vi "Match VI Names in String.vi"(10 "Application:All VIs In Memory":string[](array[string]), 11 "string":string) -> (3 "vi names":T1(array[cluster]))   [LabVIEW 2020, in "Explain Error Improved Dialog.lvlib"]
uses:
  Explain Error Improved Dialog/Explain Error Improved Dialog.lvlib
  <vilib>/regexp/Match Regular Expression.xnode
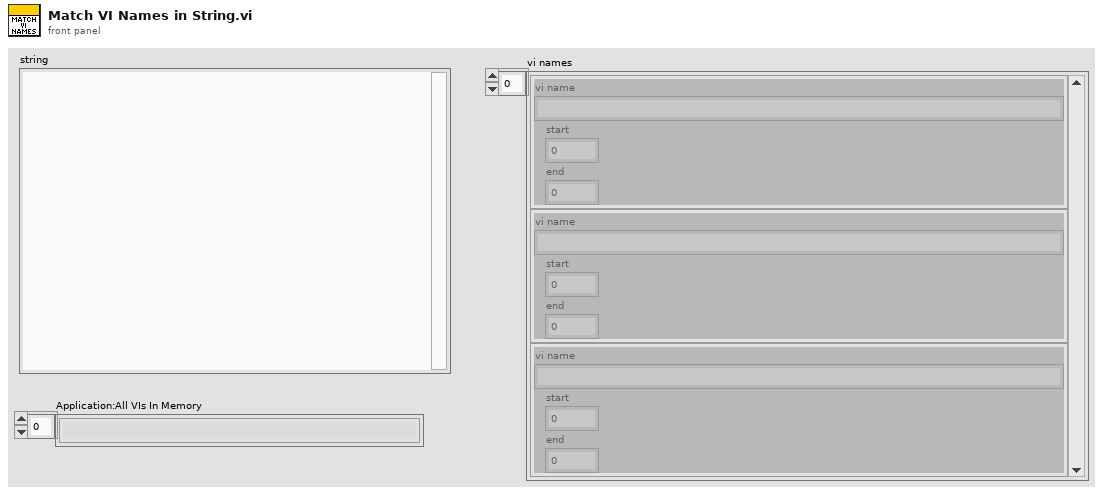
[diagram p1: front panel]
types:
  T1 = cluster{"vi name":string, "start":i32, "end":i32}[]
  T2 = cluster{"vi name":string, "start":i32, "end":i32}
  T3 = cluster{"submatch":string, "start":i32, "end":i32}
  T4 = cluster{"submatch":string, "start":i32, "end":i32}[]
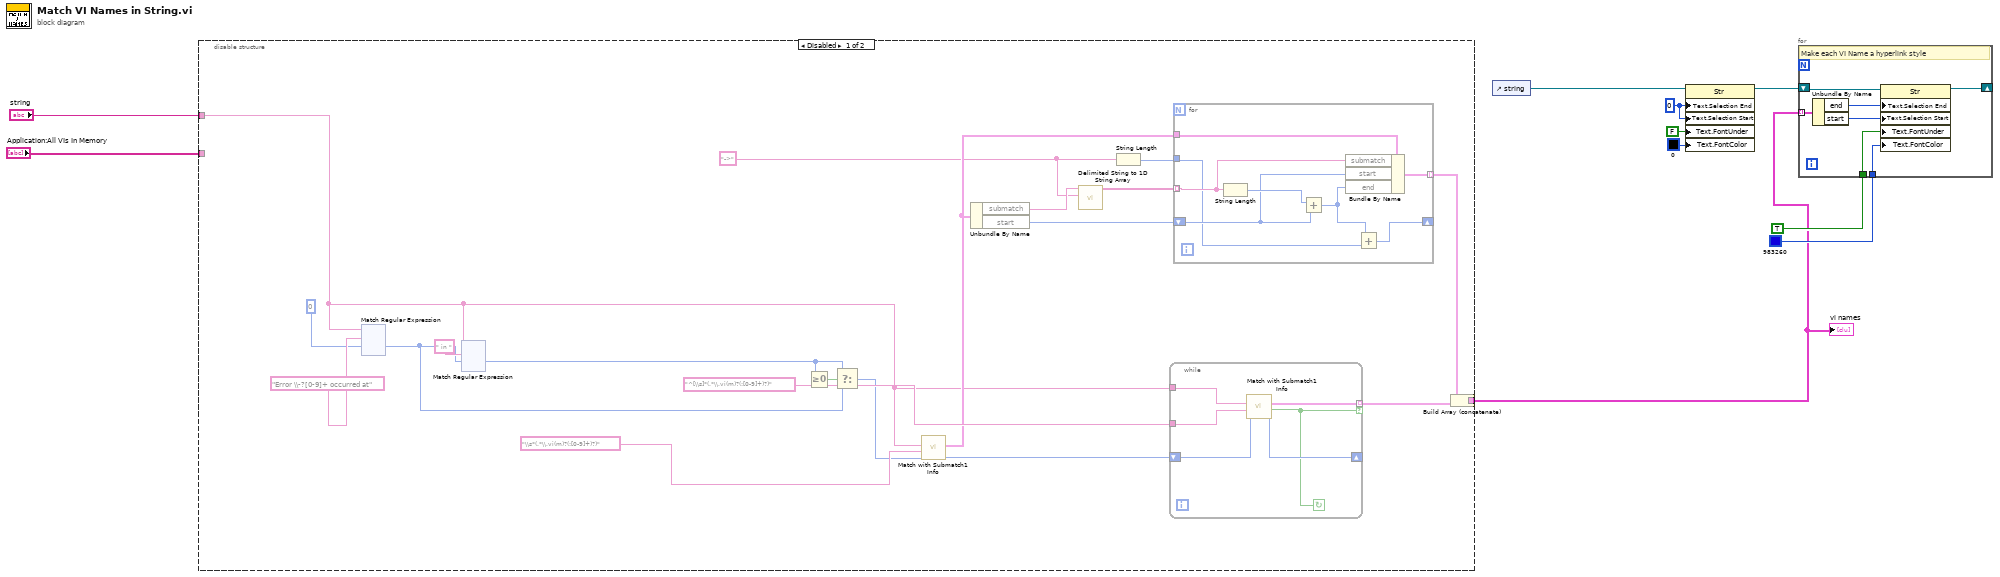
[diagram p0: block diagram]
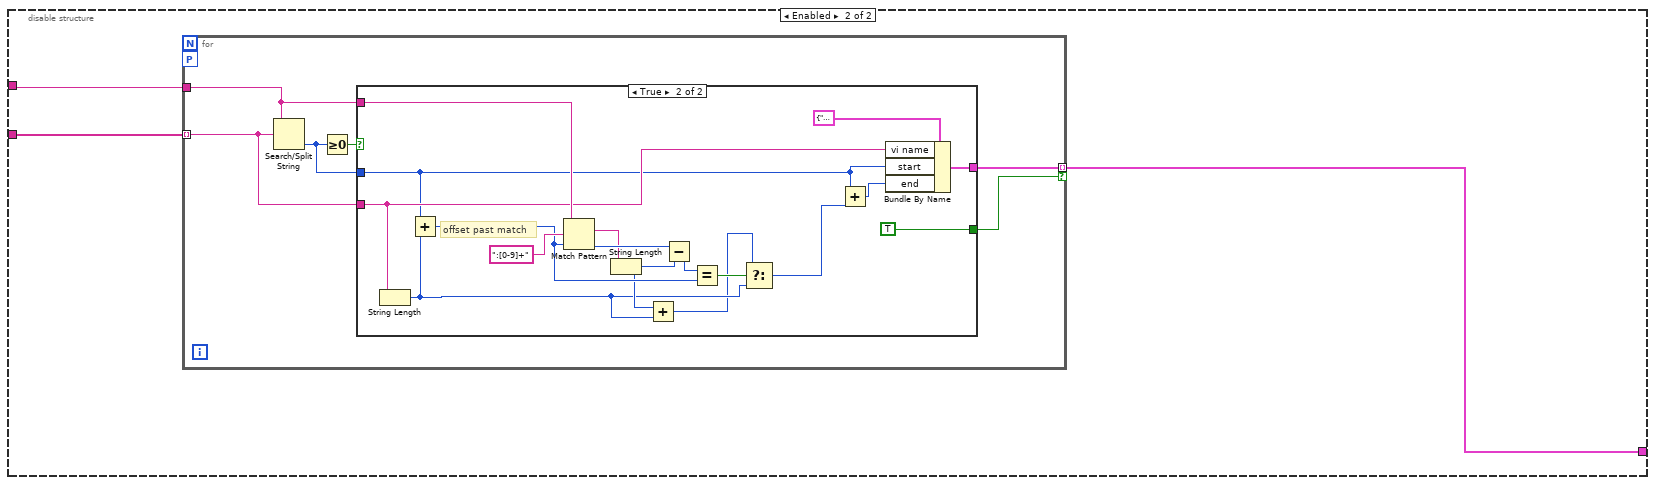
[diagram p2: hidden frame]
diagram:
  w8 = u32 0 ("Text.Selection:End")
  n1 = disable-structure shown="Disabled" {
    disable-tunnel: [w27 w273] -> w3
    disable-tunnel: "string" -> [w18 w274]
    disable-tunnel: "Application:All VIs In Memory" -> [_ w275]
    frame Disabled {
      w12 = "->" ("regular expression")
      n2 = xnode "Match Regular Expression"("input string"=w18, "regular expression"="Error \\-?[0-9]+ occurred at", "offset (0)"=0 ("offset past match in")) -> ("offset past match"=w16:i32)  [unwired: 3 in, 4 out]
      n3 = xnode "Match Regular Expression"("input string"=w18, "regular expression"=" in ", "offset (0)"=w16) -> ("offset past match"=w15:i32)  [unwired: 3 in, 4 out]
      n4 = Greater Or Equal To 0?(x=w15) -> (x >= 0?=w17:bool)
      n5 = Select(t=w15, s=w17, f=w16) -> (s? t:f=w14:i32)
      n6 = call "Match with Submatch1 Info.vi"("offset past match in"=w14, "regular expression"="\\s*(.*\\.vi(m)?(:[0-9]+)?)", "string"=w18) -> ("offset past whole match"=w22:i32, "submatch 1"=w24:T3)  [unwired: 6 in, 1 out]
      n7 = Unbundle By Name(w24) -> ("submatch"=w13:string, "start"=w25:i32)
      n8 = call <vilib>:"Delimited String to 1D String Array.vi"("delimiter"=w12, "delimited string"=w13) -> ("string array"=w11:string[])  [unwired: 9 in]
      n9 = String Length(string=w12) -> (length=w26:i32)
      n10 = while {
        tunnel: w18 -> [w272]
        tunnel: "^[\\s]*(.*\\.vi(m)?(:[0-9]+)?)" ("regular expression") -> [w271]
        shift-right: [w270] -> _
        shift-left: w22 -> [w268]
        tunnel: [w267] -> w30 mode=indexing if=w269
        stop <- w269 continue-if-true
        n11 = call "Match with Submatch1 Info.vi"("offset past match in"=w268, "regular expression"=w271, "string"=w272) -> ("offset past whole match"=w270:i32, "match found?"=w269:bool, "submatch 1"=w267:T3)  [unwired: 6 in]
      }
      n12 = for {
        tunnel: w11 -> [w264] mode=indexing
        tunnel: w26 -> [w261]
        shift-right: [w259] -> _
        shift-left: w25 -> [w263]
        tunnel: w24 -> [w265]
        tunnel: [w262] -> w23 mode=indexing
        n13 = String Length(string=w264) -> (length=w266:i32)
        n14 = Add(x=w266, y=w263) -> (x+y=w260:i32)
        n15 = Bundle By Name(cluster=w265, "submatch"=w264, "start"=w263, "end"=w260) -> (w262:T3)
        n16 = Add(x=w260, y=w261) -> (x+y=w259:i32)
      }
      n17 = Build Array (concatenate)(w23, w30) -> (w27:T4)
    }
    frame Enabled {
      n18 = for {
        tunnel: w275 -> [w281] mode=indexing
        tunnel: w274 -> [w276]
        tunnel: [w278] -> w273 mode=indexing if=w277
        workers-P: _ -> [_]
        n19 = Search/Split String(string=w276, search string/char (-)=w281) -> (offset of match=w279:i32)  [unwired: 1 in, 2 out]
        n20 = Greater Or Equal To 0?(x=w279) -> (x >= 0?=w280:bool)
        n21 = case shown="True" w280 {
          tunnel: w281 -> [_ w288]
          tunnel: w279 -> [_ w287]
          tunnel: [_ w296] -> w278
          tunnel: [_ TRUE] -> w277
          tunnel: w276 -> [_ w294]
          frame False {
          }
          frame True {
            # "offset past match"
            n22 = String Length(string=w288) -> (length=w283:i32)
            n23 = Add(x=w287, y=w283) -> (x+y=w286:i32)
            n24 = Match Pattern(string=w294, regular expression=":[0-9]+", offset (0)=w286) -> (match substring=w285:string, offset past match=w290:i32)  [unwired: 2 out]
            n25 = String Length(string=w285) -> (length=w284:i32)
            n26 = Add(x=w284, y=w283) -> (x+y=w282:i32)
            n27 = Subtract(x=w290, y=w284) -> (x-y=w292:i32)
            n28 = Equal?(x=w292, y=w286) -> (x = y?=w291:bool)
            n29 = Select(t=w282, s=w291, f=w283) -> (s? t:f=w289:i32)
            n30 = Add(x=w287, y=w289) -> (x+y=w297:i32)
            n31 = Bundle By Name(cluster=T2 {"vi name"="", "start"=0, "end"=0}, "vi name"=w288, "start"=w287, "end"=w297) -> (w296:T2)
          }
        }
      }
    }
  }
  "vi names" <- w3
  n32 = control-ref of="string"() -> (w4:refnum<vi>)
  n33 = property class="Str"(reference=w4, "Text.Selection End"=w8, "Text.Selection Start"=w8, "Text.FontUnder"=FALSE ("Text.Font:Underline"), "Text.FontColor"=u32 0 ("Text.Font:Color")) -> (reference out=w7:refnum<vi>)  [unwired: 1 in, 1 out]
  n34 = for {
    tunnel: w3 -> [w304] mode=indexing
    shift-right: [w301] -> _
    shift-left: w7 -> [w305]
    tunnel: u32 983260 -> [w300]
    tunnel: TRUE ("Text.Font:Underline") -> [w299]
    # "Make each VI Name a hyperlink style"
    n35 = Unbundle By Name(w304) -> ("end"=w303:i32, "start"=w302:i32)
    n36 = property class="Str"(reference=w305, "Text.Selection End"=w303, "Text.Selection Start"=w302, "Text.FontUnder"=w299, "Text.FontColor"=w300) -> (reference out=w301:refnum<vi>)  [unwired: 1 in, 1 out]
  }
